vi "Configure Timing (DC).vi"(0 "VISA resource name":refnum<visa-resource-name>, 5 "Period (0.05 second)":dbl=0.05 min=0.0005 max=60.0 step=0.0001 format="%^#_5g", 11 "error in (no error)":errorcluster, 12 "Measurement Delay (0.004 second)":dbl=0.004 min=5e-05 max=59.998 step=1e-06 format="%^#_5g") -> (4 "VISA resource name out":refnum<visa-resource-name>, 15 "error out":errorcluster)   [LabVIEW 2017, in "ADCMT 6240.lvlib"]
doc: "This VI configures timing for DC mode."
uses:
  ADCMT 6240.lvlib
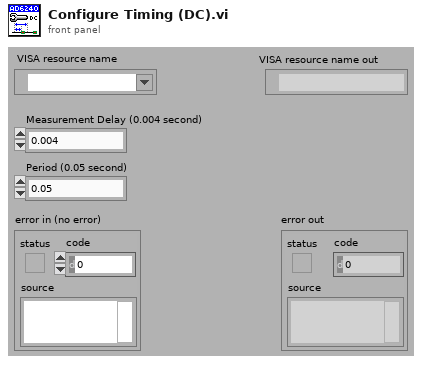
[diagram p1: front panel]
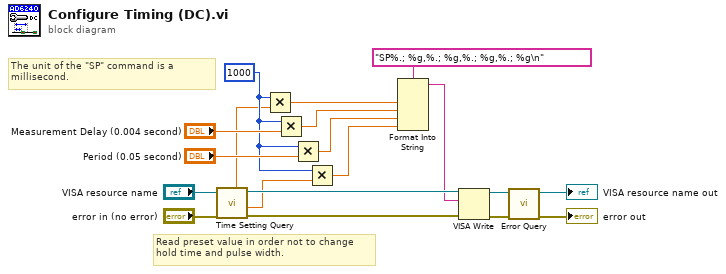
[diagram p0: block diagram]
diagram:
  w11 = 1000
  # "The unit of the \"SP\" command is a millisecond."
  # "Read preset value in order not to change hold time and pulse width."
  n1 = call "Time Setting Query.vi"("error in (no error)"="error in (no error)", "VISA resource name"="VISA resource name") -> ("error out"=w7:errorcluster, "Pulse Width (seconds)"=w1:dbl, "VISA resource name out"=w8:refnum<visa-resource-name>, "Hold Time (seconds)"=w6:dbl)  [unwired: 4 in, 2 out]
  n2 = Multiply(x=w11, y=w6) -> (x*y=w14:dbl)
  n3 = Multiply(x=w11, y="Measurement Delay (0.004 second)") -> (x*y=w3:dbl)
  n4 = Multiply(x=w11, y="Period (0.05 second)") -> (x*y=w4:dbl)
  n5 = Multiply(x=w11, y=w1) -> (x*y=w5:dbl)
  n6 = Format Into String(format string="SP%.; %g,%.; %g,%.; %g,%.; %g\n", w14, w3, w4, w5) -> (resulting string=w2:string)  [unwired: 2 in, 1 out]
  n7 = VISA Write(VISA resource name=w8, write buffer=w2, error in (no error)=w7) -> (VISA resource name out=w17:refnum<visa-resource-name>, error out=w16:errorcluster)  [unwired: 1 out]
  n8 = call "Error Query.vi"("error in (no error)"=w16, "VISA resource name"=w17) -> ("error out"=→"error out":errorcluster, "VISA resource name out"=→"VISA resource name out":refnum<visa-resource-name>)  [unwired: 6 in, 2 out]
